vi "POV to Buttons Angle.vi"(11 "POV Input":dbl) -> (0 "NE":bool, 1 "SE":bool, 2 "SW":bool, 3 "NW":bool)   [LabVIEW 2014]
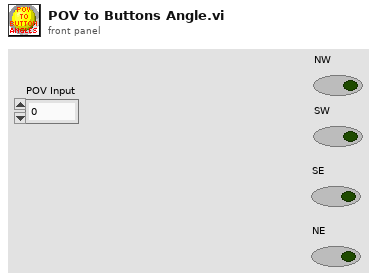
[diagram p1: front panel]
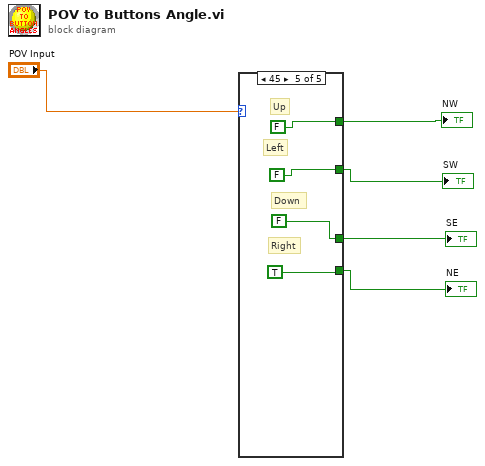
[diagram p0: block diagram]
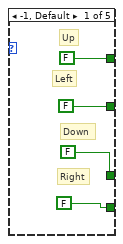
[diagram p2: hidden frame]
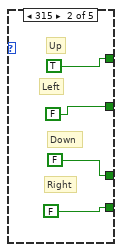
[diagram p3: hidden frame]
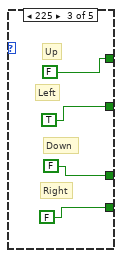
[diagram p4: hidden frame]
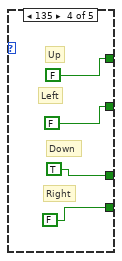
[diagram p5: hidden frame]
diagram:
  n1 = case shown="45" "POV Input" {
    tunnel: [FALSE TRUE FALSE FALSE FALSE] -> w4
    tunnel: [FALSE FALSE TRUE FALSE FALSE] -> w3
    tunnel: [FALSE FALSE FALSE FALSE TRUE] -> w1
    tunnel: [FALSE FALSE FALSE TRUE FALSE] -> w2
    frame -1, Default {
      # "Right"
      # "Down"
      # "Left"
      # "Up"
    }
    frame 315 {
      # "Right"
      # "Down"
      # "Left"
      # "Up"
    }
    frame 225 {
      # "Right"
      # "Down"
      # "Left"
      # "Up"
    }
    frame 135 {
      # "Right"
      # "Down"
      # "Left"
      # "Up"
    }
    frame 45 {
      # "Right"
      # "Down"
      # "Left"
      # "Up"
    }
  }
  "NW" <- w4
  "SW" <- w3
  "SE" <- w2
  "NE" <- w1
